vi "Init Instruments.vi"(8 "error in":errorcluster, 10 "Physical Instr CFGs":string[](array[string]), 11 "Target MSS in":refnum<class "MSS Target Actor.lvclass">) -> (0 "error out":errorcluster, 3 "Target MSS out":refnum<class "MSS Target Actor.lvclass">)   [LabVIEW 2023, in "MSS Target Actor.lvlib" / "MSS Target Actor.lvclass"]
uses:
  MSS Target Actor.lvclass
  MSS Target Actor.lvclass/MSS Target Actor.ctl
  MSS/MSS.lvclass
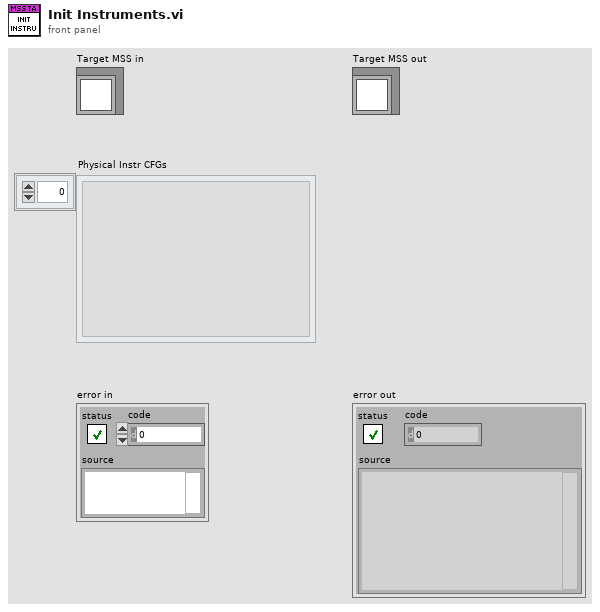
[diagram p1: front panel]
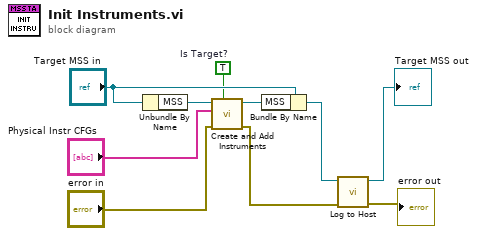
[diagram p0: block diagram]
diagram:
  w1 = TRUE  # Is Target?
  n1 = Unbundle By Name("Target MSS in") -> ("MSS"=w10:refnum<class "MSS.lvclass">)
  n2 = call "Create and Add Instruments.vi"("Is Target?"=w1, "Error In"="error in", "Instr CFGs"="Physical Instr CFGs", "MSS in"=w10) -> ("Error Out"=w4:errorcluster, "MSS out"=w8:refnum<class "MSS.lvclass">)  [unwired: 5 in, 1 out]
  n3 = Bundle By Name(cluster="Target MSS in", "MSS"=w8) -> (w3:refnum<class "MSS Target Actor.lvclass">)
  n4 = call "Log to Host.vi"("error in"=w4, "MSS Target Actor in"=w3) -> ("error out"=→"error out":errorcluster, "MSS Target Actor out"=→"Target MSS out":refnum<class "MSS Target Actor.lvclass">)  [unwired: 8 in]
